vi "String_to_Pathname.vi"(1 "Input String":string) -> (0 "path":path)   [LabVIEW 2021]
uses:
  Globals/Preference_global.vi
  Globals/Constants_global.vi
panel:
  out "dataFolder":path
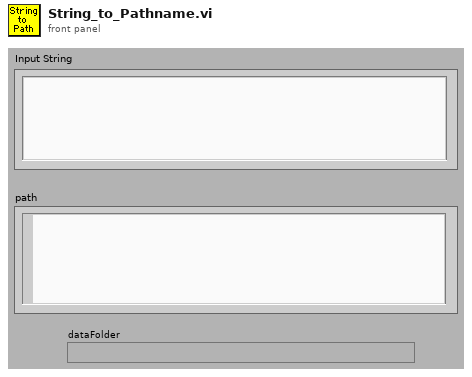
[diagram p1: front panel]
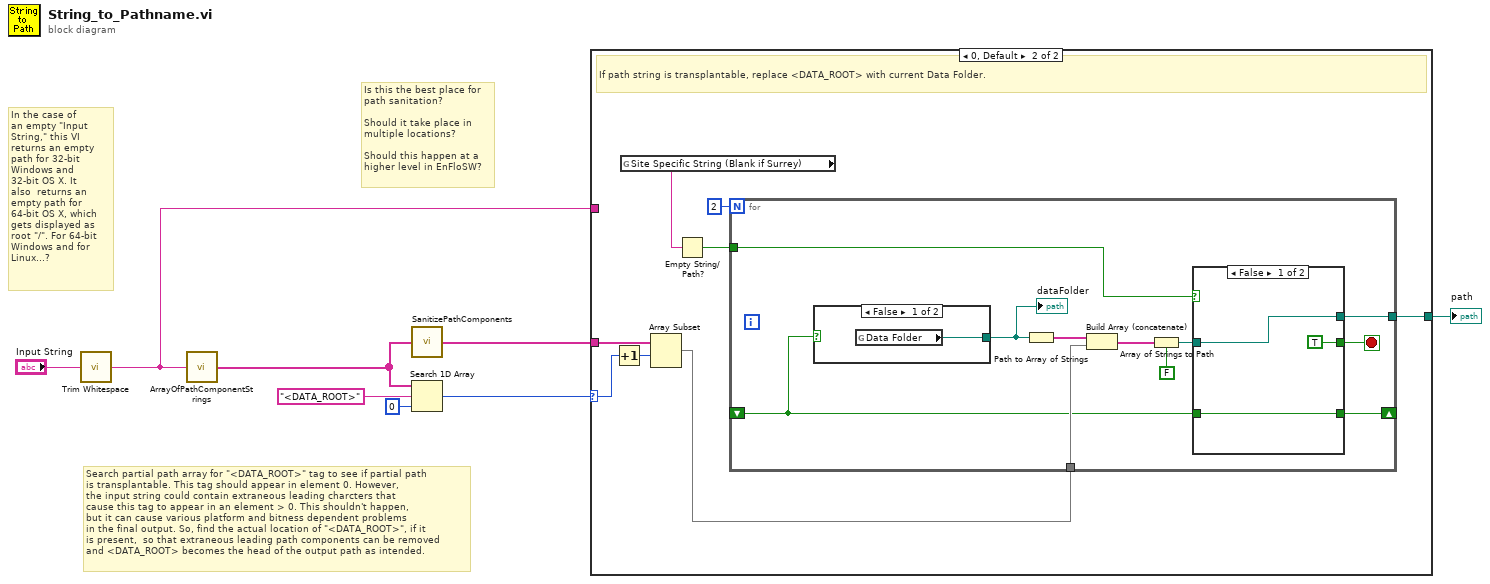
[diagram p0: block diagram]
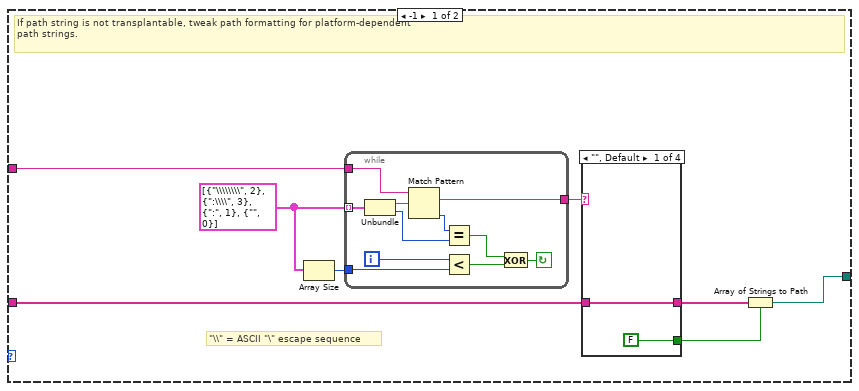
[diagram p2: hidden frame]
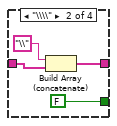
[diagram p3: hidden frame]
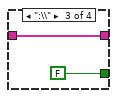
[diagram p4: hidden frame]
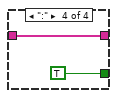
[diagram p5: hidden frame]
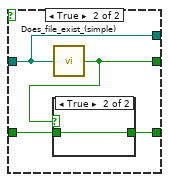
[diagram p6: hidden frame]
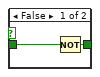
[diagram p7: hidden frame]
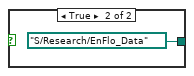
[diagram p8: hidden frame]
diagram:
  # "Is this the best place for\npath sanitation?\n\nShould it take place in\nmultiple locations?\n\nShould this happen at a\nhigher level in EnFloSW?"
  # "In the case of \nan empty \"Input \nString,\" this VI \nreturns an empty\npath for 32-bit\nWindows and\n32-bit OS X. It\nalso  returns an\nempty path for \n64-bit OS X, which\ngets displayed as\nroot \"/\". For 64-bit \nWindows and for\nLinux...?"
  # "Search partial path array for \"<DATA_ROOT>\" tag to see if partial path\nis transplantable. This tag should appear in element 0. However,\nthe input string could contain extraneous leading charcters that \ncause this tag to appear in an element > 0. This shouldn't happen,\nbut it can cause various platform and bitness dependent problems\nin the final output. So, find the actual location of \"<DATA_ROOT>\", if it\nis present,  so that extraneous leading path components can be removed\nand <DATA_ROOT> becomes the head of the output path as intended."
  n1 = call <vilib>:"Trim Whitespace.vi"("string"="Input String") -> ("trimmed string"=w7:string)  [unwired: 1 in]
  n2 = call "ArrayOfPathComponentStrings.vi"("PathStringIn"=w7) -> ("ArrayOfPathComponentStringsOut"=w3:string[])
  n3 = call "SanitizePathComponents.vi"("PathComponentsIn"=w3) -> ("SanitizedComponentsOut"=w4:string[])
  n4 = Search 1D Array(1D array=w3, element="<DATA_ROOT>", start index (0)=0) -> (index of element=w2:i32)
  n5 = case shown="0, Default" w2 {
    selector: w2 -> [_ w43]
    tunnel: w4 -> [w12 w44]
    tunnel: w7 -> [w14 _]
    tunnel: [w9 w40] -> w1
    frame -1 {
      w15 = cluster{string, i32}[] [{"\\\\\\\\", 2}, {":\\\\", 3}, {":", 1}, {"", 0}]
      # "\"\\\\\" = ASCII \"\\\" escape sequence"
      # "If path string is not transplantable, tweak path formatting for platform-dependent\npath strings."
      n6 = Array Size(array=w15) -> (size(s)=w16:i32)
      n7 = while {
        tunnel: w15 -> [w29] mode=indexing
        tunnel: w16 -> [w37]
        tunnel: [w32] -> w13
        tunnel: w14 -> [w30]
        i -> [w31]
        stop <- w33 continue-if-true
        n8 = Unbundle(w29) -> (w27:string, w28:i32)
        n9 = Match Pattern(string=w30, regular expression=w27) -> (match substring=w32:string, offset past match=w35:i32)  [unwired: 1 in, 2 out]
        n10 = Equal?(x=w35, y=w28) -> (x = y?=w34:bool)
        n11 = Less?(x=w31, y=w37) -> (x < y?=w36:bool)
        n12 = Exclusive Or(1:w36, 2:w34) -> (0:w33:bool)
      }
      n13 = case shown="\"\", Default" w13 {
        tunnel: [FALSE FALSE FALSE TRUE] -> w11
        tunnel: w12 -> [w18 w19 w23 w25]
        tunnel: [w18 w20 w23 w25] -> w10
        frame "", Default {
        }
        frame "\\\\" {
          n14 = Build Array (concatenate)("\\", w19) -> (w20:string[])
        }
        frame ":\\" {
        }
        frame ":" {
        }
      }
      n15 = Array of Strings to Path(0:w10, 1:w11) -> (2:w9:path)
    }
    frame 0, Default {
      # "If path string is transplantable, replace <DATA_ROOT> with current Data Folder."
      n16 = Increment(x=w43) -> (x+1=w45:i32)
      n17 = global read "Preference_global.vi" "Site Specific String (Blank if Surrey)"() -> (w42:string)
      n18 = Array Subset(array=w44, index=w45) -> (w41:string[])  [unwired: 1 in]
      n19 = Empty String/Path?(string/path=w42) -> (empty?=w38:bool)
      n20 = for {
        N: 2 -> [_]
        tunnel: w41 -> [w54]
        tunnel: [w49] -> w40
        tunnel: w38 -> [w46]
        shift-right: [w48] -> _
        shift-left: _ -> [w47]
        stop <- w50 stop-if-true
        n21 = case shown="False" w47 {
          tunnel: [w67 path "S:/Research/EnFlo_Data" ("Path")] -> w56
          frame False {
            n22 = global read "Constants_global.vi" "Data Folder"() -> (w67:path)
          }
          frame True {
          }
        }
        "dataFolder" <- w56
        n23 = Path to Array of Strings(0:w56) -> (2:w55:string[])  [unwired: 1 out]
        n24 = Build Array (concatenate)(w55, w54) -> (w53:string[])
        n25 = Array of Strings to Path(0:w53, 1:FALSE) -> (2:w51:path)
        n26 = case shown="False" w46 {
          tunnel: w51 -> [w59 w63]
          tunnel: [TRUE ("exists?") w62] -> w50
          tunnel: [w59 w63] -> w49
          tunnel: [w57 w61] -> w48
          tunnel: w47 -> [w57 w60]
          frame False {
          }
          frame True {
            n27 = call "Does_file_exist_(simple).vi"("Pathname"=w63) -> ("exists?"=w62:bool)
            n28 = case shown="True" w62 {
              tunnel: [w65 w66] -> w61
              tunnel: w60 -> [w64 w66]
              frame False {
                n29 = Not(x=w64) -> (.not. x?=w65:bool)
              }
              frame True {
              }
            }
          }
        }
      }
    }
  }
  "path" <- w1
